vi "RunTest2.vi"(8 "error in (no error)":errorcluster, 11 "AjustesPrevios in":refnum<class "AjustesPrevios.lvclass">) -> (0 "error out":errorcluster, 2 "resultado":string, 3 "AjustesPrevios out":refnum<class "AjustesPrevios.lvclass">)   [LabVIEW 2019]
uses:
  AjustesPrevios.lvclass
  <vilib>/Utility/miscctls.llb/LVRowAndColumnTypeDef.ctl
  Controles/MessageAjustesPrev.ctl
  Prueba/Prueba.lvclass
  Controles/EstadosAjsutesPrev.ctl
  Globals/globales.vi
  Instrumento/Pistofono/Pistofono.lvclass
  QMH/User Event - Stop/User Event - Stop.lvlib
  QMH/Message Queue/Message Queue.lvlib
  QMH/Message Queue/Enqueue Message (Single).vi
  Controles/ClusterLecturaPistofono.ctl
  Controles/ClusterLecturaKeithley.ctl
  RerenceAllControlsToolkit/_get control reference by name.vi
  RerenceAllControlsToolkit/_get mutiple control reference by name.vi
  D:/REPO/GitHub/procal/Pruebas/Prueba/Prueba.lvclass
  Prueba04/Control/Slide.ctl
  Prueba04/Prueba04.lvclass
panel:
  in  "generar_CAM 2":bool
  out "Sim":bool
  out "Vguardado":dbl
  out "size_frec":i32
  in  "Tabs":enum32{"Ajustes 1", "Ajustes 2", "Ajustes 3"}(tab)
  out "factor_correccion_enviado":dbl format="%#.5g"
  in  "aplicar FC":bool
  out "Voltaje mV":dbl format="%#.3g"
  out "Nivel Medido":dbl format="%#.2g"
  out "temperatura":dbl
  out "presion":dbl
  in  "humedad":dbl
  out "nivel_emitido":dbl
  out "factor_correccion":dbl format="%#.5g"
  in  "siguiente1":bool
  in  "Sensibilidad":dbl(knob)=0.1 scale=0.01..1.0 scale format="%#_6p"
  out "voltaje a CAM":dbl format="%#_5g"
  out "frecuencia":dbl
  in  "guardar":bool
  in  "generar":bool
  in  "anterior2":bool
  in  "ajusteAmp(mV)":T1=1.0 caption="Ajuste de amplitud [V]" scale=0.1..1.5
  in  "siguiente2":bool
  in  "generar_CAM":bool
  out "voltaje":dbl format="%_3g"
  out "frecuencia":dbl
  out "NPS":dbl format="%#_4g"
  in  "anterior3":bool
  in  "terminar":bool
  out "Tabla":string[][](table)
  # "Información Pistófono"
  # "Nivel Medido [dB]"
  # "Factor de Corrección Calculado"
  # "Factor de Corrección Enviado"
  # "Voltaje [V]"
  # "Temperatura [°C]"
  # "Presión [hPa]"
  # "Humedad [%]"
  # "Nivel Emitido [dB]"
  # "Ajuste Previo 1 : Igualación de Patrones"
  # "Monitoreo"
  # "Voltaje a CAM"
  # "V"
  # "Frecuencia"
  # "Hz"
  # "Ajuste Previo 2 : Ajuste Acústico Emisor Multitono"
  # "Monitoreo"
  # "NPS"
  # "dB"
  # "Voltaje a CAM"
  # "V"
  # "Frecuencia"
  # "Hz"
  # "Ajuste Previo 3 : Niveles de Presión Sonora de Referencia"
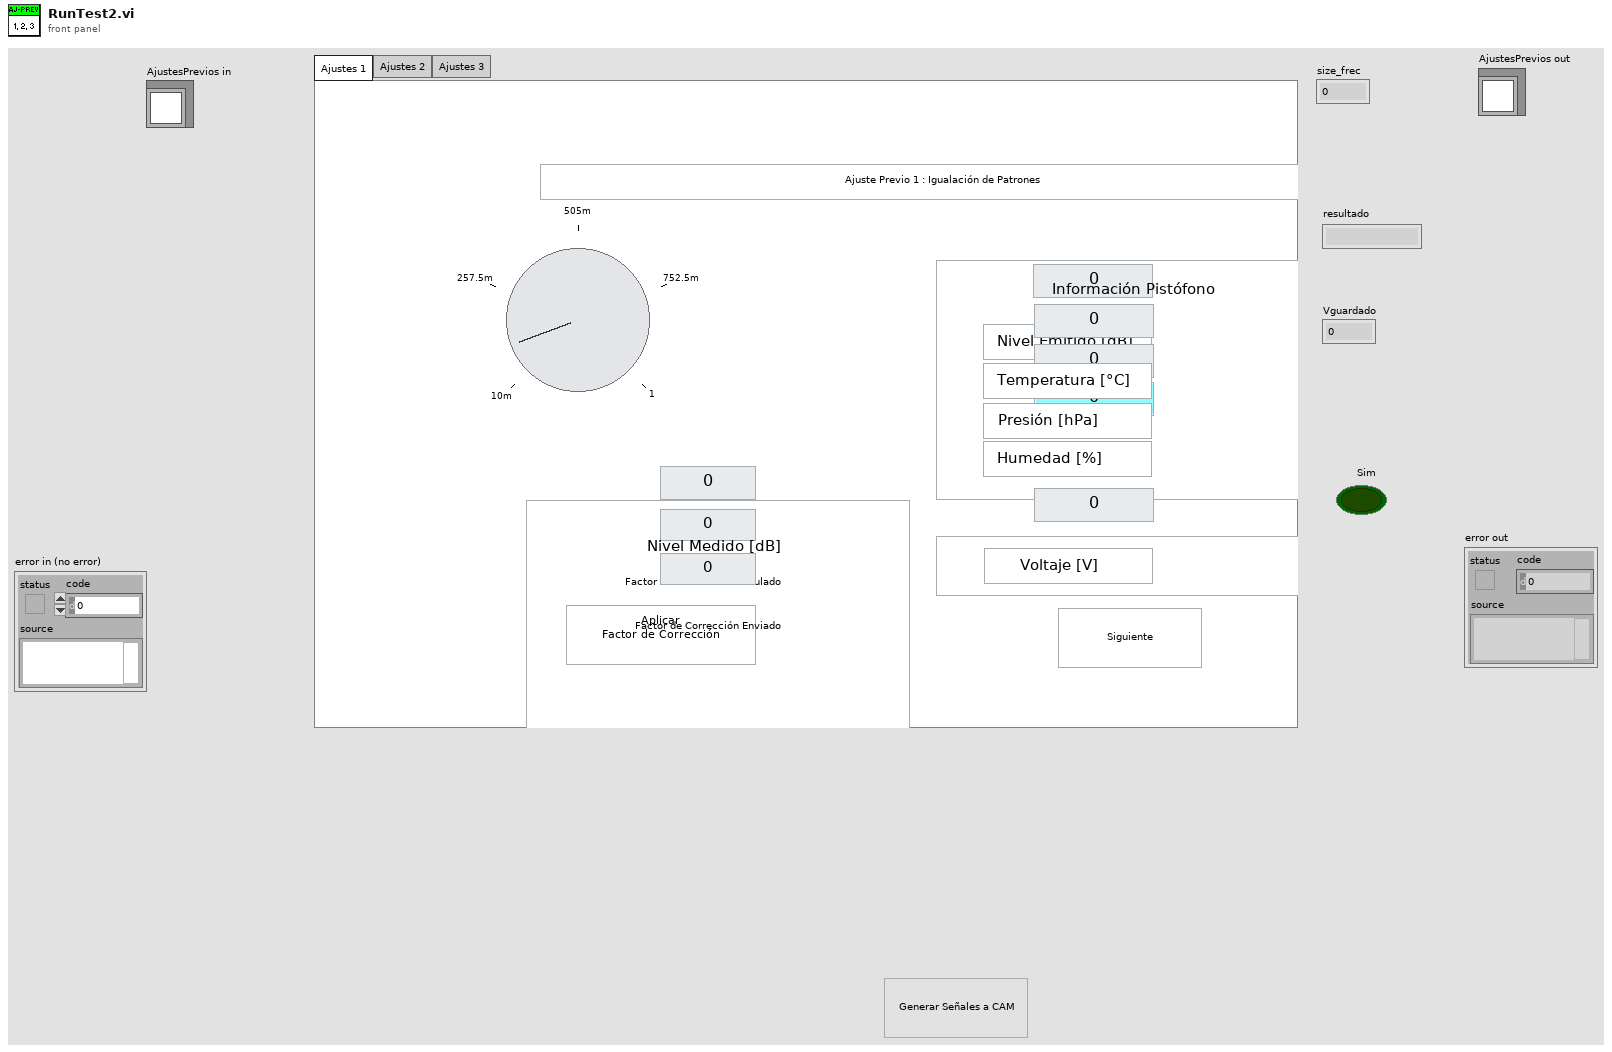
[diagram p1: front panel]
types:
  T1 = typedef "Prueba04.lvclass/Slide.ctl" = dbl
  T2 = typedef "Prueba.lvclass/MessageAjustesPrev.ctl" = cluster{"Estados":T3, "Data":variant}
  T3 = typedef "Prueba.lvclass/EstadosAjsutesPrev.ctl" = enum16{"inicio", "iniciaInstrumentos", "configurarTabla", "Ajustes1", "escribeSensib", "aplicarFC", "escribir_datos_igual_patrones", "preguntar_gen", "Ajustes2", "generar", "detenerGEN", "monitorear", "guardar", "Ajustes3", "generarCAM_94", "avisoParaCAM114", "generarCAM_114", "salir", "error", "reconec_pistofono"}
  T4 = typedef "LVRowAndColumnTypeDef.ctl" = cluster{"Row":i32, "Column":i32}
  T5 = typedef "Message Queue.lvlib/All Message Queues.ctl" = cluster{"MHL":refnum<queue>, "Inst_CNT90":refnum<queue>, "Inst_DS360":refnum<queue>, "Inst_Keithley2002":refnum<queue>, "Inst_DAQ":refnum<queue>, "BD":refnum<queue>, "Pistofono":refnum<queue>, "Nexus":refnum<queue>}
  T6 = typedef "AjustesPrevios.lvclass/ClusterLecturaPistofono.ctl" = cluster{"temperatura":dbl, "presion":dbl, "nivel_emitido":dbl}
  T7 = typedef "AjustesPrevios.lvclass/ClusterLecturaKeithley.ctl" = cluster{"Nivel_Medido_dB":dbl, "voltaje_mV":dbl}
  T8 = enum8{"Enabled", "Disabled", "Disabled and Grayed Out"}
  T9 = cluster{"ControlName":string, "ControlReference":refnum<vi>}[]
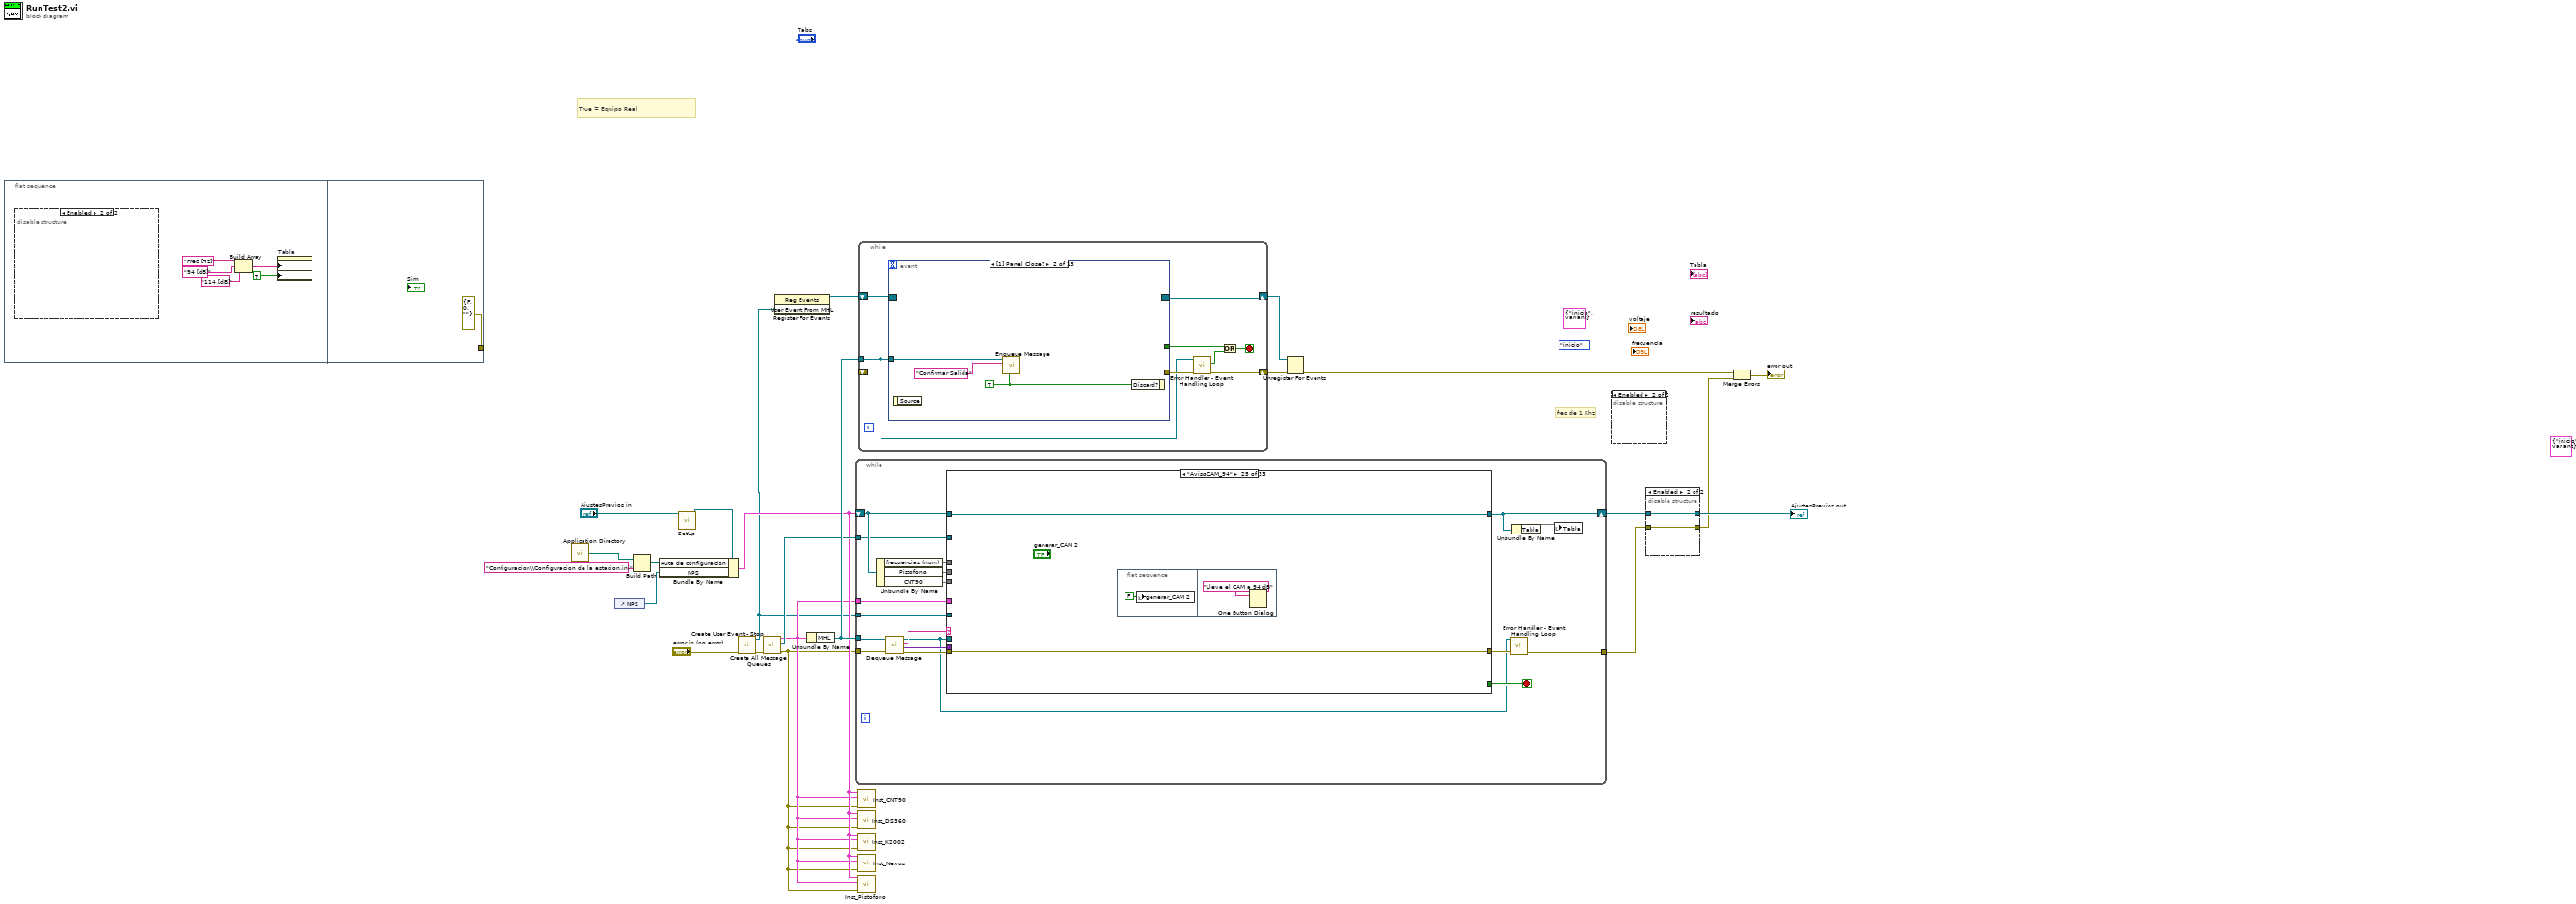
[diagram p0: block diagram]
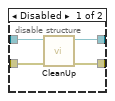
[diagram p2: hidden frame]
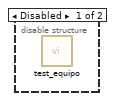
[diagram p3: hidden frame]
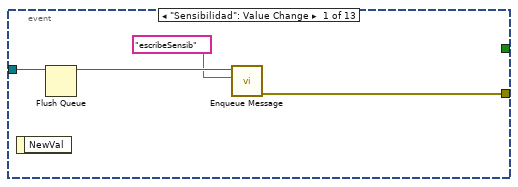
[diagram p4: hidden frame]
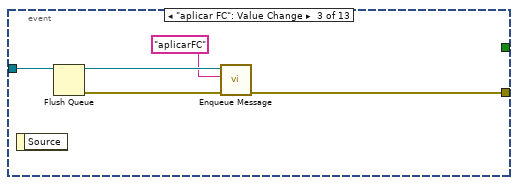
[diagram p5: hidden frame]
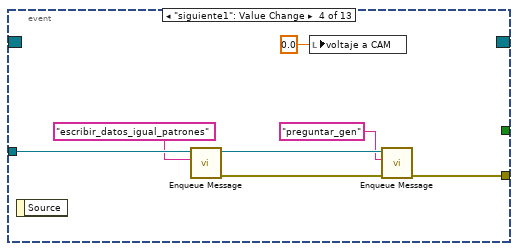
[diagram p6: hidden frame]
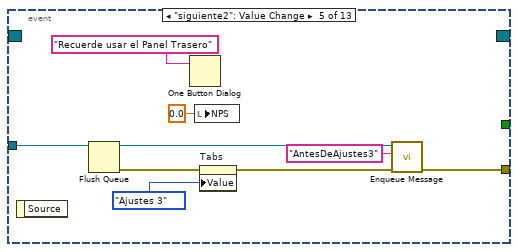
[diagram p7: hidden frame]
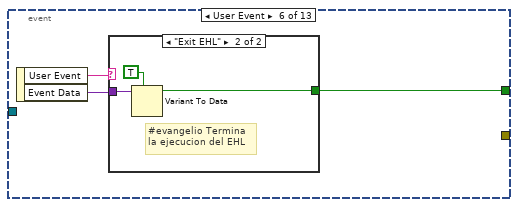
[diagram p8: hidden frame]
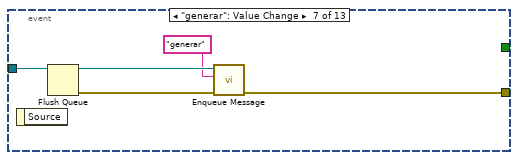
[diagram p10: hidden frame]
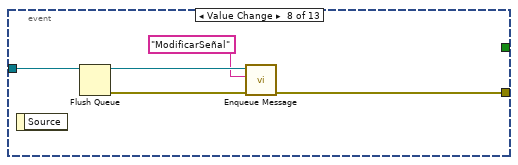
[diagram p11: hidden frame]
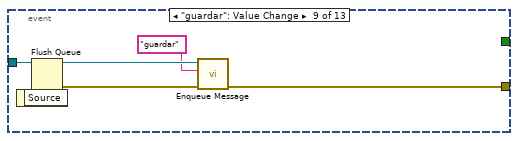
[diagram p12: hidden frame]
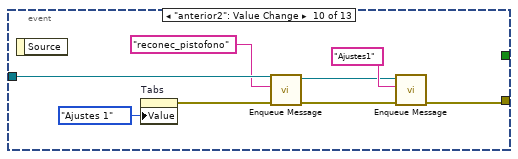
[diagram p13: hidden frame]
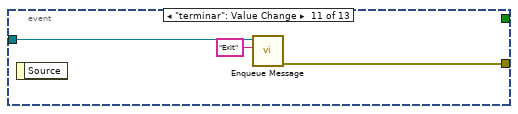
[diagram p14: hidden frame]
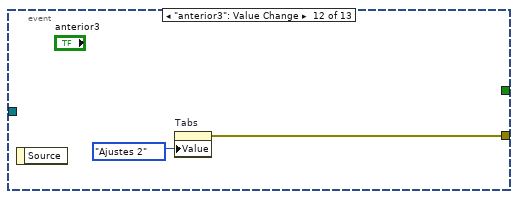
[diagram p15: hidden frame]
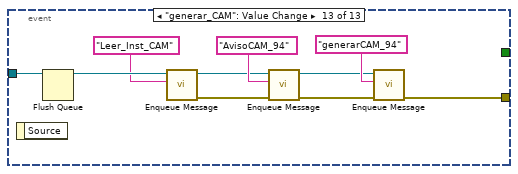
[diagram p16: hidden frame]
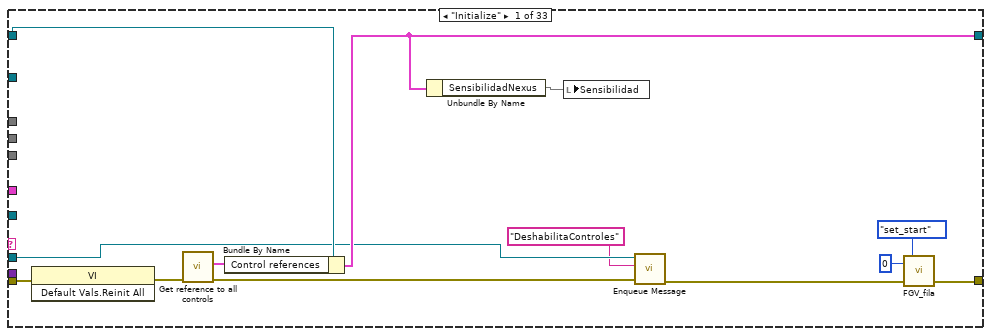
[diagram p17: hidden frame]
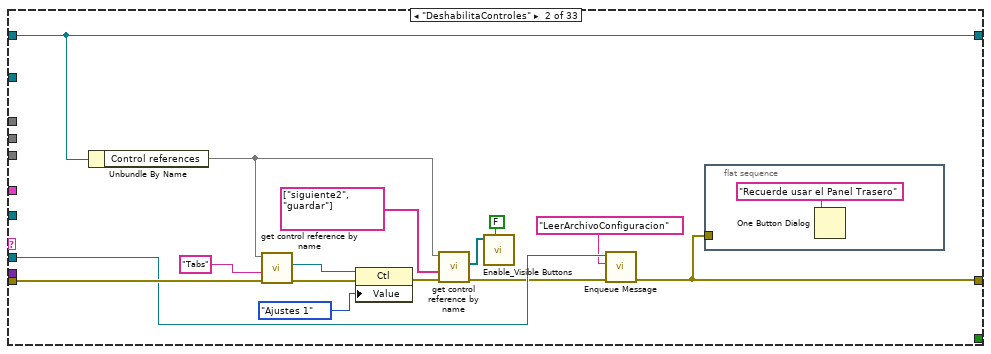
[diagram p18: hidden frame]
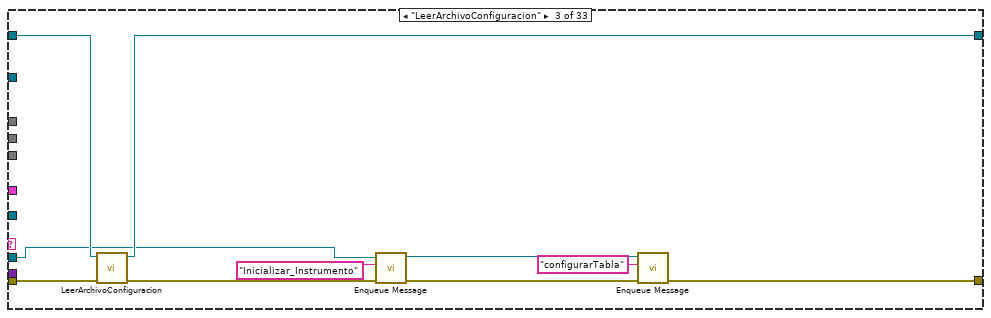
[diagram p19: hidden frame]
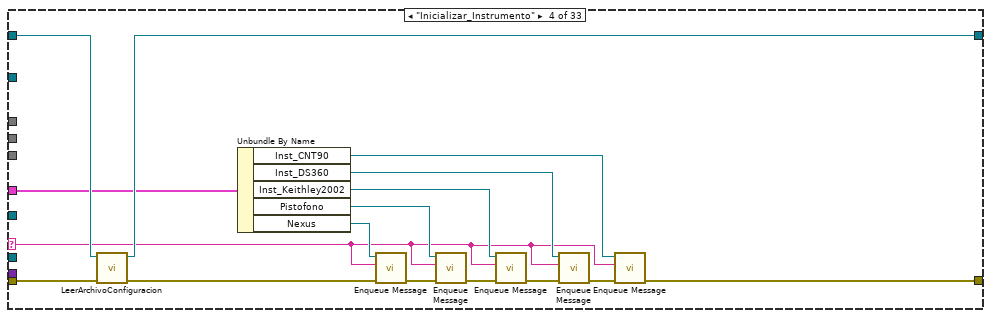
[diagram p20: hidden frame]
diagram:
  (unwired) T2 {"Estados"=enum."inicio", "Data"=variant}
  (unwired) EstadosAjsutesPrev."inicio" ("Estados")
  (unwired) T2 {"Estados"=enum."inicio", "Data"=variant}
  # "frec de 1 Khz"
  # "True = Equipo Real"
  n1 = flat-sequence {
    tunnel: [errorcluster {"status"=FALSE, "code"=0, "source"=""} ("error in (no error)")] -> _
    frame #0 {
      n2 = disable-structure shown="Enabled" {
        frame Disabled {
          n3 = Bundle By Name(cluster=T4 {"Row"=0, "Column"=0} ("Active Cell:Active Cell"), "Row"=-2, "Column"=-2) -> (w29:T4)
          n4 = property on="Tabla" class="Tbl (strict)"("Active Cell"=w29, "CellFontSize"=u32 20 ("Active Cell:Cell Font:Size"), "Justify"=enum16{"Left", "Center", "Right"}."Center" ("Active Cell:Cell Justification")) -> ()  [unwired: 2 in, 2 out]
        }
        frame Enabled {
        }
      }
    }
    frame #1 {
      n5 = Build Array("Frec [Hz]", "94 [dB]", "114 [dB]" ("element")) -> (w31:string[])
      n6 = property on="Tabla" class="Tbl (strict)"("Column Headers[]"=w31, "Col Headers Vis"=TRUE ("Visible Items:Column Headers Visible")) -> ()  [unwired: 2 in, 2 out]
    }
    frame #2 {
    }
  }
  n7 = call <vilib>:"Application Directory.vi"() -> ("Application Directory"=w13:path)
  n8 = control-ref of="NPS"() -> (w1:refnum<vi>)
  n9 = Build Path(base path=w13, name or relative path="Configuracion\\Configuracion de la estacion.ini") -> (appended path=w12:path)
  n10 = call-dynamic "SetUp.vi"("AjustesPrevios in"="AjustesPrevios in") -> ("AjustesPrevios out"=w11:refnum<class "AjustesPrevios.lvclass">)  [unwired: 9 in, 1 out]
  n11 = Bundle By Name(cluster=w11, "Ruta de configuracion"=w12, "NPS"=w1) -> (w7:cluster{})
  n12 = call "Create User Event - Stop.vi"("error in (no error)"="error in (no error)") -> ("error out"=w15:errorcluster, "User Event From MHL"=w5:refnum<user-event>)  [unwired: 9 in]
  n13 = call "Create All Message Queues.vi"("error in (no error)"=w15) -> ("error out"=w2:errorcluster, "PL Queues Array"=w8:refnum<queue>[], "All Message Queues out"=w6:T5)  [unwired: 8 in]
  n14 = register-events(w5) -> (reference out=w19:refnum<event-registration>)  [unwired: 2 in, 1 out]
  n15 = Unbundle By Name(w6) -> ("MHL"=w9:refnum<queue>)
  n16 = while {
    tunnel: w9 -> [w46]
    tunnel: w2 -> [w45]
    shift-right: [w51] -> w20
    shift-left: w7 -> [w52]
    tunnel: w6 -> [w41]
    tunnel: w8 -> [w40]
    tunnel: w5 -> [w39]
    tunnel: [w36] -> w4
    stop <- w53 stop-if-true
    n17 = Unbundle By Name(w52) -> ("frecuencias (num)"=w48, "Pistofono"=w49, "CNT90"=w47)
    n18 = call "Dequeue Message.vi"("error in (no error)"=w45, "Message Queue"=w46) -> ("error out"=w44:errorcluster, "Message Data"=w42:variant, "Message"=w43:string, "dup Message Queue"=w37:refnum<queue>)  [unwired: 6 in]
    n19 = case shown="\"AvisoCAM_94\"" w43 {
      selector: w43 -> [_ _ _ w93 w109 _ _ _ _ _ _ _ _ _ _ _ _ _ _ _ _ _ _ _ _ _ _ _ w425 _ _ _ _]
      tunnel: w44 -> [w61 w80 w91 w107 w121 w133 w136 w161 w163 w170 w179 w185 w196 w208 w212 w230 w247 w268 w270 w286 w293 w303 w305 w311 w313 w325 w370 w394 w428 w445 w454 w456 w458]
      tunnel: [w66 w67 w87 w92 w108 w123 w135 w155 w163 w167 w175 w183 w191 w205 w211 w219 w248 w264 w270 w275 w288 w299 w305 w309 w313 w337 w366 w390 w421 w439 w452 w456 w458] -> w38
      tunnel: [_ _ _ _ _ _ _ _ _ _ _ _ _ _ _ _ _ _ _ _ _ _ _ _ _ _ _ _ w423 _ _ _ _] -> w53
      tunnel: w52 -> [w59 w81 w89 w105 w120 w132 w142 w158 w162 w171 w180 w186 w194 w209 w216 w229 w239 w267 w269 w281 w289 w302 w304 w310 w312 w331 w369 w386 w424 w448 w453 w455 w457]
      tunnel: [w58 w81 w88 w104 w120 w132 w142 w156 w162 w171 w180 w186 w195 w200 w217 w237 w238 w267 w269 w281 w289 w298 w304 w310 w312 w328 w369 w383 w424 w448 w453 w455 w457] -> w51
      tunnel: w49 -> [_ _ _ _ _ _ _ _ _ _ _ _ _ _ _ _ _ _ _ _ _ _ _ _ _ _ _ _ _ _ _ _ _]
      tunnel: w48 -> [_ _ _ _ _ _ _ _ _ _ _ _ _ _ _ _ _ _ _ _ _ _ _ _ _ w334 _ w387 _ _ _ _ _]
      tunnel: w47 -> [_ _ _ _ _ _ _ _ _ _ _ _ _ _ _ _ _ _ _ _ _ _ _ _ _ _ _ _ _ _ _ _ _]
      tunnel: w37 -> [w57 w70 w86 _ _ _ w137 w153 _ _ _ _ _ _ _ _ w243 _ _ _ _ _ _ _ _ w323 w368 w373 w427 w441 _ _ _]
      tunnel: w42 -> [_ _ _ _ _ _ _ _ _ _ w178 w184 _ w207 _ _ _ _ _ _ _ _ _ _ _ _ _ _ _ w444 _ _ _]
      tunnel: w41 -> [_ _ _ w103 w119 w131 _ _ _ w169 _ _ w190 _ w215 w228 _ w266 _ w285 w292 w296 _ w308 _ w321 _ w377 _ _ w451 _ _]
      tunnel: w40 -> [_ _ _ _ _ _ _ _ _ _ _ _ _ _ _ _ _ _ _ _ _ _ _ _ _ _ _ _ w422 _ _ _ _]
      tunnel: w39 -> [_ _ _ _ _ _ _ _ _ _ _ _ _ _ _ _ _ _ _ _ _ _ _ _ _ _ _ _ w426 _ _ _ _]
      frame "Initialize" {
        n20 = invoke class="VI" method="Default Vals.Reinit All"(error in=w61) -> (error out=w62:errorcluster)  [unwired: 2 in, 2 out]
        n21 = call "Get reference to all controls.vi"("error in (no error)"=w62) -> ("error out"=w55:errorcluster, "Control references"=w60:T9)  [unwired: 5 in]
        n22 = Bundle By Name(cluster=w59, "Control references"=w60) -> (w58:cluster{})
        n23 = Unbundle By Name(w58) -> ("SensibilidadNexus"=w63)
        n24 = local write "Sensibilidad"(w63) -> ()
        n25 = call-poly "Enqueue Message.vi"("error in (no error)"=w55, "Message"="DeshabilitaControles", "Message Queue"=w57) -> ("error out"=w54:errorcluster)  [unwired: 7 in, 1 out]
        n26 = call "FGV_fila.vi"("error in (no error)"=w54, "fila_inicial"=0, "action"=enum16{"increment", "set_start", "get"}."set_start") -> ("error out"=w66:errorcluster)  [unwired: 1 in, 1 out]
      }
      frame "DeshabilitaControles" {
        n27 = Unbundle By Name(w81) -> ("Control references"=w71)
        n28 = call-poly "get control reference by name.vi"("error in (no error)"=w80, "Control name"="Tabs", "Control references"=w71) -> ("error out"=w78:errorcluster, "Ctl Refnum"=w75:refnum<vi>)  [unwired: 3 in]
        n29 = property on="Property Node" class="Ctl"(reference=w75, error in=w78, "Value"=enum32{"Ajustes 1", "Ajustes 2", "Ajustes 3"}."Ajustes 1" ("Tabs")) -> (error out=w77:errorcluster)  [unwired: 1 out]
        n30 = call-poly "get control reference by name.vi"("error in (no error)"=w77, "Control names"=string[] ["siguiente2", "guardar"] ("Control name"), "Control references"=w71) -> ("error out"=w69:errorcluster, "References"=w72:refnum<vi>[])  [unwired: 3 in]
        n31 = call "Enable_Visible Buttons.vi"("Enable? (T)"=FALSE, "Controls Ref Array"=w72) -> ()  [unwired: 10 in]
        n32 = call-poly "Enqueue Message.vi"("error in (no error)"=w69, "Message"="LeerArchivoConfiguracion", "Message Queue"=w70) -> ("error out"=w67:errorcluster)  [unwired: 7 in, 1 out]
        n33 = flat-sequence {
          tunnel: w67 -> [_]
          frame #0 {
            n34 = One Button Dialog(message="Recuerde usar el Panel Trasero") -> ()  [unwired: 1 in, 1 out]
          }
        }
      }
      frame "LeerArchivoConfiguracion" {
        n35 = call "LeerArchivoConfiguracion.vi"("error in"=w91, "AjustesPrevios in"=w89) -> ("error out"=w90:errorcluster, "AjustesPrevios out"=w88:refnum<class "AjustesPrevios.lvclass">)  [unwired: 8 in]
        n36 = call-poly "Enqueue Message.vi"("error in (no error)"=w90, "Message"="Inicializar_Instrumento", "Message Queue"=w86) -> ("error out"=w87:errorcluster, "dup Message Queue"=w84:refnum<queue>)  [unwired: 7 in]
        n37 = call-poly "Enqueue Message.vi"("Message"="configurarTabla", "Message Queue"=w84) -> ()  [unwired: 8 in, 2 out]
      }
      frame "Inicializar_Instrumento" {
        n38 = call "LeerArchivoConfiguracion.vi"("error in"=w107, "AjustesPrevios in"=w105) -> ("error out"=w106:errorcluster, "AjustesPrevios out"=w104:refnum<class "AjustesPrevios.lvclass">)  [unwired: 8 in]
        n39 = Unbundle By Name(w103) -> ("Inst_CNT90"=w98:refnum<queue>, "Inst_DS360"=w97:refnum<queue>, "Inst_Keithley2002"=w96:refnum<queue>, "Pistofono"=w95:refnum<queue>, "Nexus"=w94:refnum<queue>)
        n40 = call-poly "Enqueue Message.vi"("error in (no error)"=w106, "Message"=w93, "Message Queue"=w94) -> ("error out"=w102:errorcluster)  [unwired: 7 in, 1 out]
        n41 = call-poly "Enqueue Message.vi"("error in (no error)"=w102, "Message"=w93, "Message Queue"=w95) -> ("error out"=w101:errorcluster)  [unwired: 7 in, 1 out]
        n42 = call-poly "Enqueue Message.vi"("error in (no error)"=w101, "Message"=w93, "Message Queue"=w96) -> ("error out"=w100:errorcluster)  [unwired: 7 in, 1 out]
        n43 = call-poly "Enqueue Message.vi"("error in (no error)"=w100, "Message"=w93, "Message Queue"=w97) -> ("error out"=w99:errorcluster)  [unwired: 7 in, 1 out]
        n44 = call-poly "Enqueue Message.vi"("error in (no error)"=w99, "Message"=w93, "Message Queue"=w98) -> ("error out"=w92:errorcluster)  [unwired: 7 in, 1 out]
      }
      frame "Detener_Instrumento" {
        n45 = Unbundle By Name(w119) -> ("Inst_CNT90"=w114:refnum<queue>, "Inst_DS360"=w113:refnum<queue>, "Inst_Keithley2002"=w112:refnum<queue>, "Pistofono"=w111:refnum<queue>, "Nexus"=w110:refnum<queue>)
        n46 = call-poly "Enqueue Message.vi"("error in (no error)"=w121, "Message"=w109, "Message Queue"=w110) -> ("error out"=w118:errorcluster)  [unwired: 7 in, 1 out]
        n47 = call-poly "Enqueue Message.vi"("error in (no error)"=w118, "Message"=w109, "Message Queue"=w111) -> ("error out"=w117:errorcluster)  [unwired: 7 in, 1 out]
        n48 = call-poly "Enqueue Message.vi"("error in (no error)"=w117, "Message"=w109, "Message Queue"=w112) -> ("error out"=w116:errorcluster)  [unwired: 7 in, 1 out]
        n49 = call-poly "Enqueue Message.vi"("error in (no error)"=w116, "Message"=w109, "Message Queue"=w113) -> ("error out"=w115:errorcluster)  [unwired: 7 in, 1 out]
        n50 = call-poly "Enqueue Message.vi"("error in (no error)"=w115, "Message"=w109, "Message Queue"=w114) -> ("error out"=w108:errorcluster)  [unwired: 7 in, 1 out]
      }
      frame "Detener_Instrumento_Final" {
        w122 = "Detener_Instrumento"
        # "No consideramos el pistofono\nporque ya fue desconectado"
        n51 = Unbundle By Name(w131) -> ("Inst_CNT90"=w127:refnum<queue>, "Inst_DS360"=w126:refnum<queue>, "Inst_Keithley2002"=w125:refnum<queue>, "Nexus"=w124:refnum<queue>)  [unwired: 1 out]
        n52 = call-poly "Enqueue Message.vi"("error in (no error)"=w133, "Message"=w122, "Message Queue"=w124) -> ("error out"=w130:errorcluster)  [unwired: 7 in, 1 out]
        n53 = call-poly "Enqueue Message.vi"("error in (no error)"=w130, "Message"=w122, "Message Queue"=w125) -> ("error out"=w129:errorcluster)  [unwired: 7 in, 1 out]
        n54 = call-poly "Enqueue Message.vi"("error in (no error)"=w129, "Message"=w122, "Message Queue"=w126) -> ("error out"=w128:errorcluster)  [unwired: 7 in, 1 out]
        n55 = call-poly "Enqueue Message.vi"("error in (no error)"=w128, "Message"=w122, "Message Queue"=w127) -> ("error out"=w123:errorcluster)  [unwired: 7 in, 1 out]
      }
      frame "Confirmar Salida" {
        n56 = Two Button Dialog(message="¿Quieres cerrar la aplicación?", 1:"No" ("T button name (\"OK\")"), 2:"Si" ("T button name (\"OK\")")) -> (T button?=w138:bool)
        n57 = case shown="True" w138 {
          tunnel: w136 -> [w143 w151]
          tunnel: [w143 w146] -> w135
          tunnel: w137 -> [_ w149]
          tunnel: "Detener_Instrumento" ("Message") -> [_ w147]
          frame False {
          }
          frame True {
            n58 = call-poly "Enqueue Message.vi"("Priority Message? (F)"=TRUE, "error in (no error)"=w151, "Message"=w147, "Message Queue"=w149) -> ("error out"=w150:errorcluster, "dup Message Queue"=w145:refnum<queue>)  [unwired: 6 in]
            n59 = call-poly "Enqueue Message.vi"("error in (no error)"=w150, "Message"="Exit", "Message Queue"=w145) -> ("error out"=w146:errorcluster)  [unwired: 7 in, 1 out]
          }
        }
      }
      frame "configurarTabla" {
        n60 = call-poly "Enqueue Message.vi"("error in (no error)"=w161, "Message"="Ajustes1", "Message Queue"=w153) -> ("error out"=w155:errorcluster)  [unwired: 7 in, 1 out]
        n61 = Unbundle By Name(w158) -> ("Tabla"=w160, "frecuencias"=w154)
        n62 = call "escribeEnTabla.vi"("parametros"=w154, "col"=0, "tabla in"=w160) -> ("tabla out"=w157:string[][])  [unwired: 8 in]
        n63 = Bundle By Name(cluster=w158, "Tabla"=w157) -> (w156:cluster{})
      }
      frame "--------------------------Ajustes 1---------------------------" {
      }
      frame "Ajustes1" {
        w164 = "Leer_Instrumento" ("Message")
        n64 = Unbundle By Name(w169) -> ("Pistofono"=w166:refnum<queue>, "Inst_Keithley2002"=w165:refnum<queue>)
        n65 = call-poly "Enqueue Message.vi"("error in (no error)"=w170, "Message"=w164, "Message Queue"=w165) -> ("error out"=w168:errorcluster)  [unwired: 7 in, 1 out]
        n66 = call-poly "Enqueue Message.vi"("error in (no error)"=w168, "Message"=w164, "Message Queue"=w166) -> ("error out"=w167:errorcluster)  [unwired: 7 in, 1 out]
      }
      frame "DatoRecibidoPistofono" {
        n67 = Variant To Data(error in=w179, type=T6 {"temperatura"=0.0, "presion"=0.0, "nivel_emitido"=0.0} ("clusterPistofono"), Variant=w178) -> (data=w176:T6, error out=w175:errorcluster)
        n68 = Unbundle By Name(w176) -> ("temperatura"=→"temperatura":dbl, "presion"=→"presion":dbl, "nivel_emitido"=→"nivel_emitido":dbl)
      }
      frame "DatoRecibidoCNT90" {
        n69 = Variant To Data(error in=w185, type=0.0, Variant=w184) -> (data=→"frecuencia":dbl, error out=w183:errorcluster)
      }
      frame "aplicarFC" {
        n70 = Unbundle By Name(w190) -> ("Nexus"=w189:refnum<queue>)
        n71 = local read "factor_correccion"() -> (w188:dbl)
        "factor_correccion_enviado" <- w188
        n72 = Unbundle By Name(w194) -> ("igualacion_de_patrones"=w193)
        n73 = Bundle By Name(cluster=w193, "FactorCorreccionSensNexus"=w188) -> (w192:cluster{})
        n74 = call-poly "Enqueue Message.vi"("error in (no error)"=w196, "Message Data"=w188, "Message"="AplicarFactorCorreccion", "Message Queue"=w189) -> ("error out"=w191:errorcluster)  [unwired: 6 in, 1 out]
        n75 = Bundle By Name(cluster=w194, "igualacion_de_patrones"=w192) -> (w195:cluster{})
      }
      frame "DatoRecibidoK2002" {
        n76 = Variant To Data(error in=w208, type=T7 {"Nivel_Medido_dB"=0.0, "voltaje_mV"=0.0} ("K2002 Data Cluster"), Variant=w207) -> (data=w202:T7, error out=w206:errorcluster)
        n77 = Unbundle By Name(w202) -> ("voltaje_mV"=w198:dbl, "Nivel_Medido_dB"=w197:dbl)
        "Voltaje mV" <- w198
        "Nivel Medido" <- w197
        "voltaje a CAM" <- w198
        "NPS" <- w197
        n78 = local read "nivel_emitido"() -> (w204:dbl)
        n79 = call "FactorCorreccion.vi"("error in (no error)"=w206, "Nivel Medido"=w197, "Nivel Emitido"=w204) -> ("error out"=w205:errorcluster, "factor_correccion"=→"factor_correccion":dbl)  [unwired: 7 in]
        n80 = Bundle By Name(cluster=w209, "Voltaje enviado a CAM"=w198, "Humedad"="humedad") -> (w200:cluster{})
      }
      frame "escribeSensib" {
        n81 = local read "Sensibilidad"() -> (w210:dbl)
        n82 = Unbundle By Name(w215) -> ("Nexus"=w214:refnum<queue>)
        n83 = call-poly "Enqueue Message.vi"("error in (no error)"=w212, "Message Data"=w210, "Message"="EscribirSensibilidad", "Message Queue"=w214) -> ("error out"=w211:errorcluster)  [unwired: 6 in, 1 out]
        n84 = Bundle By Name(cluster=w216, "SensibilidadNexus"=w210) -> (w217:cluster{})
      }
      frame "escribir_datos_igual_patrones" {
        w221 = "No_Leer_Instrumento" ("Message")
        n85 = Unbundle By Name(w228) -> ("Inst_Keithley2002"=w222:refnum<queue>, "Inst_CNT90"=w224:refnum<queue>, "Inst_DS360"=w226:refnum<queue>, "Pistofono"=w227:refnum<queue>)
        n86 = call-poly "Enqueue Message.vi"("error in (no error)"=w230, "Message"="Detener_Instrumento", "Message Queue"=w227) -> ("error out"=w225:errorcluster)  [unwired: 7 in, 1 out]
        n87 = call-poly "Enqueue Message.vi"("error in (no error)"=w225, "Message"=w221, "Message Queue"=w226) -> ("error out"=w223:errorcluster)  [unwired: 7 in, 1 out]
        n88 = call-poly "Enqueue Message.vi"("error in (no error)"=w223, "Message"=w221, "Message Queue"=w224) -> ("error out"=w220:errorcluster)  [unwired: 7 in, 1 out]
        n89 = call-poly "Enqueue Message.vi"("error in (no error)"=w220, "Message"=w221, "Message Queue"=w222) -> ("error out"=w219:errorcluster)  [unwired: 7 in, 1 out]
        n90 = Unbundle By Name(w229) -> ("igualacion_de_patrones"=w236)
        n91 = local read "nivel_emitido"() -> (w235:dbl)
        n92 = local read "temperatura"() -> (w234:dbl)
        n93 = local read "humedad"() -> (w232:dbl)
        n94 = local read "presion"() -> (w233:dbl)
        n95 = Bundle By Name(cluster=w236, "Nivel Emitido Pistófono [dB]"=w235, "Temperatura interna Pistófono[ºC]"=w234, "Presión Medida Pistófono  [hPa]"=w233, "Humedad Relativa Aire [%]"=w232) -> (w231:cluster{})
        n96 = Bundle By Name(cluster=w229, "igualacion_de_patrones"=w231) -> (w237:cluster{})
      }
      frame "preguntar_gen" {
        # "Escribe en Archivo INI"
        n97 = Flush Queue(queue=w243, error in (no error)=w247) -> (queue out=w244:refnum<queue>, error out=w245:errorcluster)  [unwired: 1 out]
        n98 = call "selccionaGenerador.vi"("error in (no error)"=w245) -> ("error out"=w246:errorcluster, "Generador"=w241:string)  [unwired: 1 in]
        n99 = call "EscribirArchivoConfiguracion.vi"("error in"=w246, "TipoGenerador"=w241, "AjustesPrevios in"=w239) -> ("error out"=w242:errorcluster, "TipoGenerador out"=w240:string, "AjustesPrevios out"=w238:refnum<class "AjustesPrevios.lvclass">)  [unwired: 6 in]
        n100 = case shown="\"Externo\", Default" w240 {
          tunnel: [w250 w256] -> w248
          tunnel: w242 -> [w254 w257]
          tunnel: w244 -> [w255 _]
          frame "Interno" {
            n101 = call-poly "Enqueue Message.vi"("error in (no error)"=w254, "Message"="Detener_Instrumento", "Message Queue"=w255) -> ("error out"=w251:errorcluster, "dup Message Queue"=w252:refnum<queue>)  [unwired: 7 in]
            n102 = call-poly "Enqueue Message.vi"("error in (no error)"=w251, "Message"="Exit", "Message Queue"=w252) -> ("error out"=w250:errorcluster)  [unwired: 7 in, 1 out]
          }
          frame "Externo", Default {
            n103 = local read "ajusteAmp(mV)"() -> (w259:T1)
            n104 = property on="Tabs" class="TabCtl (strict)"(error in=w257, "Value"=enum32{"Ajustes 1", "Ajustes 2", "Ajustes 3"}."Ajustes 2" ("Tabs")) -> (error out=w256:errorcluster)  [unwired: 1 in, 1 out]
            n105 = One Button Dialog(message="Recuerde usar el Panel Delantero") -> ()  [unwired: 1 in, 1 out]
            n106 = local write "voltaje a CAM"(w259) -> ()
          }
        }
      }
      frame "AntesDeAjustes3" {
        w261 = "No_Leer_Instrumento" ("Message")
        n107 = Unbundle By Name(w266) -> ("Inst_CNT90"=w262:refnum<queue>, "Inst_Keithley2002"=w263:refnum<queue>)
        n108 = call-poly "Enqueue Message.vi"("error in (no error)"=w268, "Message"=w261, "Message Queue"=w263) -> ("error out"=w265:errorcluster)  [unwired: 7 in, 1 out]
        n109 = call-poly "Enqueue Message.vi"("error in (no error)"=w265, "Message"=w261, "Message Queue"=w262) -> ("error out"=w264:errorcluster)  [unwired: 7 in, 1 out]
      }
      frame "--------------------------Ajustes 2---------------------------" {
      }
      frame "generar" {
        w271 = "Leer_Instrumento" ("Message")
        n110 = Unbundle By Name(w281) -> ("Control references"=w280)
        n111 = call-poly "get control reference by name.vi"("error in (no error)"=w286, "Control name"="guardar", "Control references"=w280) -> ("error out"=w282:errorcluster, "Ctl Refnum"=w277:refnum<vi>)  [unwired: 3 in]
        n112 = property class="Ctl"(reference=w277, error in=w282, "DisabledEnum"=T8."Enabled" ("Disabled")) -> (error out=w278:errorcluster)  [unwired: 1 out]
        n113 = Unbundle By Name(w285) -> ("Inst_CNT90"=w272:refnum<queue>, "Inst_Keithley2002"=w273:refnum<queue>, "Inst_DS360"=w284:refnum<queue>)
        n114 = local read "ajusteAmp(mV)"() -> (w283:T1)
        n115 = call-poly "Enqueue Message.vi"("error in (no error)"=w278, "Message Data"=w283, "Message"="GenerarSeñal", "Message Queue"=w284) -> ("error out"=w275:errorcluster)  [unwired: 6 in, 1 out]
        n116 = call-poly "Enqueue Message.vi"("Message"=w271, "Message Queue"=w273) -> ()  [unwired: 8 in, 2 out]
        n117 = call-poly "Enqueue Message.vi"("Message"=w271, "Message Queue"=w272) -> ()  [unwired: 8 in, 2 out]
      }
      frame "ModificarSeñal" {
        n118 = local read "ajusteAmp(mV)"() -> (w290:T1)
        n119 = Unbundle By Name(w292) -> ("Inst_DS360"=w291:refnum<queue>)
        n120 = call-poly "Enqueue Message.vi"("error in (no error)"=w293, "Message Data"=w290, "Message"="GenerarSeñal", "Message Queue"=w291) -> ("error out"=w288:errorcluster)  [unwired: 6 in, 1 out]
      }
      frame "guardar" {
        n121 = Unbundle By Name(w296) -> ("Inst_DS360"=w295:refnum<queue>)
        n122 = property on="siguiente2" class="Bool"("DisabledEnum"=T8."Enabled" ("Disabled")) -> ()  [unwired: 2 in, 2 out]
        n123 = One Button Dialog(message="Voltaje guardado") -> ()  [unwired: 1 in, 1 out]
        n124 = call-poly "Enqueue Message.vi"("error in (no error)"=w303, "Message"="Detener_Instrumento", "Message Queue"=w295) -> ("error out"=w299:errorcluster)  [unwired: 7 in, 1 out]
        n125 = local read "voltaje a CAM"() -> (w297:dbl)
        "Vguardado" <- w297
        n126 = Bundle By Name(cluster=w302, "Voltaje enviado a CAM"=w297) -> (w298:cluster{})
        n127 = global write "globales.vi" "Vguardado"(w297) -> ()
      }
      frame "--------------------------Ajustes 3---------------------------" {
      }
      frame "Leer_Inst_CAM" {
        n128 = Unbundle By Name(w308) -> ("Inst_Keithley2002"=w307:refnum<queue>)
        n129 = call-poly "Enqueue Message.vi"("error in (no error)"=w311, "Message"="Leer_Instrumento", "Message Queue"=w307) -> ("error out"=w309:errorcluster)  [unwired: 7 in, 1 out]
      }
      frame "AvisoCAM_94" {
        n130 = flat-sequence {
          frame #0 {
            n131 = local write "generar_CAM 2"(FALSE ("generar_CAM")) -> ()
          }
          frame #1 {
            n132 = One Button Dialog(message="Lleve el CAM a 94 dB") -> ()  [unwired: 1 in, 1 out]
          }
        }
      }
      frame "generarCAM_94" {
        # "Envía set point a generador"
        n133 = call "FGV_fila.vi"("action"=enum16{"increment", "set_start", "get"}."get") -> ("fila out"=w330:i32)  [unwired: 3 in, 1 out]
        n134 = Unbundle By Name(w321) -> ("Inst_DS360"=w320:refnum<queue>)
        n135 = Array Size(array=w334) -> (size(s)=→"size_frec":i32)
        n136 = Index Array(array=w334, index=w330) -> (element=w324)
        n137 = local read "Vguardado"() -> (w318:dbl)
        n138 = local write "frecuencia"(w324) -> ()
        n139 = call-poly "Enqueue Message.vi"("error in (no error)"=w325, "Message Data"=w318, "Message"="GenerarSeñal", "Message Queue"=w320) -> ("error out"=w322:errorcluster)  [unwired: 6 in, 1 out]
        n140 = call "Time Delay"("error in (no error)"=w322, "Delay Time (s)"=2.0) -> ("error out"=w317:errorcluster)  [unwired: 9 in]
        n141 = while {
          tunnel: w317 -> [w361]
          tunnel: [w361] -> w339
          tunnel: w331 -> [w355]
          tunnel: w330 -> [w357]
          tunnel: [w356] -> w329
          tunnel: [w355] -> w327
          i -> [w364]
          stop <- w362 stop-if-true
          # "col"
          n142 = Unbundle By Name(w355) -> ("Tabla"=w359)
          n143 = local read "NPS"() -> (w354:dbl)
          n144 = local write "generar_CAM"(TRUE ("generar_CAM")) -> ()
          n145 = Greater?(x=w364, y=2) -> (0:w362:bool)
          n146 = call "escribeEnTablaUnValor.vi"("element"=w354, "fila"=w357, "col"=1, "tabla in"=w359) -> ("tabla out"=w356:string[][])  [unwired: 7 in]
          n147 = Wait (ms)(milliseconds to wait=u32 1000) -> ()  [unwired: 1 out]
        }
        n148 = local read "size_frec"() -> (w332:i32)
        n149 = call "FGV_fila.vi"("error in (no error)"=w339, "action"=enum16{"increment", "set_start", "get"}."increment") -> ("error out"=w338:errorcluster, "fila out"=w335:i32)  [unwired: 2 in]
        n150 = Bundle By Name(cluster=w327, "Tabla"=w329) -> (w328:cluster{})
        n151 = Greater Or Equal?(x=w335, y=w332) -> (x >= y?=w336:bool)
        n152 = local read "Vguardado"() -> (w326:dbl)
        n153 = case shown="True" w336 {
          tunnel: w338 -> [w346 w353]
          tunnel: [w345 w352] -> w337
          tunnel: w323 -> [w342 w347]
          frame False {
            n154 = local write "generar_CAM"(FALSE ("generar_CAM")) -> ()
            n155 = call-poly "Enqueue Message.vi"("error in (no error)"=w346, "Message"="generarCAM_94", "Message Queue"=w342) -> ("error out"=w345:errorcluster)  [unwired: 7 in, 1 out]
          }
          frame True {
            n156 = local write "NPS"(0.0 ("NPS")) -> ()
            n157 = call "FGV_fila.vi"("fila_inicial"=0, "action"=enum16{"increment", "set_start", "get"}."set_start") -> ()  [unwired: 2 in, 2 out]
            n158 = call-poly "Enqueue Message.vi"("error in (no error)"=w353, "Message"="avisoParaCAM114", "Message Queue"=w347) -> ("error out"=w352:errorcluster)  [unwired: 7 in, 1 out]
          }
        }
        n159 = local write "voltaje"(w326) -> ()
      }
      frame "avisoParaCAM114" {
        n160 = call-poly "Enqueue Message.vi"("error in (no error)"=w370, "Message"="generarCAM_114", "Message Queue"=w368) -> ("error out"=w366:errorcluster)  [unwired: 7 in, 1 out]
        n161 = flat-sequence {
          tunnel: w366 -> [_]
          frame #0 {
            n162 = local write "generar_CAM"(FALSE ("generar_CAM")) -> ()
            n163 = One Button Dialog(message="Lleve el CAM a 114 dB") -> ()  [unwired: 1 in, 1 out]
          }
        }
      }
      frame "generarCAM_114" {
        n164 = call "FGV_fila.vi"("action"=enum16{"increment", "set_start", "get"}."get") -> ("fila out"=w385:i32)  [unwired: 3 in, 1 out]
        n165 = local read "Vguardado"() -> (w375:dbl)
        n166 = Index Array(array=w387, index=w385) -> (element=w379)
        n167 = Unbundle By Name(w377) -> ("Inst_DS360"=w374:refnum<queue>)
        n168 = local write "frecuencia"(w379) -> ()
        n169 = call-poly "Enqueue Message.vi"("error in (no error)"=w394, "Message Data"=w375, "Message"="GenerarSeñal", "Message Queue"=w374) -> ("error out"=w378:errorcluster)  [unwired: 6 in, 1 out]
        n170 = while {
          tunnel: w378 -> [w416]
          tunnel: [w416] -> w392
          tunnel: w386 -> [w410]
          tunnel: w385 -> [w412]
          tunnel: [w411] -> w384
          tunnel: [w410] -> w382
          i -> [w419]
          stop <- w417 stop-if-true
          # "col"
          n171 = Unbundle By Name(w410) -> ("Tabla"=w414)
          n172 = local write "generar_CAM"(TRUE ("generar_CAM")) -> ()
          n173 = local read "NPS"() -> (w409:dbl)
          n174 = Greater?(x=w419, y=2) -> (0:w417:bool)
          n175 = call "escribeEnTablaUnValor.vi"("element"=w409, "fila"=w412, "col"=2, "tabla in"=w414) -> ("tabla out"=w411:string[][])  [unwired: 7 in]
          n176 = Wait (ms)(milliseconds to wait=u32 1000) -> ()  [unwired: 1 out]
        }
        n177 = local read "size_frec"() -> (w381:i32)
        n178 = call "FGV_fila.vi"("error in (no error)"=w392, "action"=enum16{"increment", "set_start", "get"}."increment") -> ("error out"=w391:errorcluster, "fila out"=w388:i32)  [unwired: 2 in]
        n179 = Bundle By Name(cluster=w382, "Tabla"=w384) -> (w383:cluster{})
        n180 = Greater Or Equal?(x=w388, y=w381) -> (x >= y?=w389:bool)
        n181 = case shown="True" w389 {
          tunnel: w391 -> [w400 w408]
          tunnel: [w399 w403] -> w390
          tunnel: w373 -> [w396 w402]
          frame False {
            n182 = local write "generar_CAM"(FALSE ("generar_CAM")) -> ()
            n183 = call-poly "Enqueue Message.vi"("error in (no error)"=w400, "Message"="generarCAM_114", "Message Queue"=w396) -> ("error out"=w399:errorcluster)  [unwired: 7 in, 1 out]
          }
          frame True {
            n184 = call "FGV_fila.vi"("fila_inicial"=0, "action"=enum16{"increment", "set_start", "get"}."set_start") -> ()  [unwired: 2 in, 2 out]
            n185 = One Button Dialog(message="Generación de frecuencias OK") -> ()  [unwired: 1 in, 1 out]
            n186 = local write "generar_CAM"(FALSE) -> ()
            n187 = call-poly "Enqueue Message.vi"("error in (no error)"=w408, "Message"="Detener_Instrumento_Final", "Message Queue"=w402) -> ("error out"=w403:errorcluster)  [unwired: 7 in, 1 out]
          }
        }
        n188 = local read "Vguardado"() -> (w380:dbl)
        n189 = local write "voltaje"(w380) -> ()
      }
      frame "Exit" {
        w423 = TRUE
        # "#evangelio Manda a cerrar el EHL"
        # "#evangelio Manda a cerrar todos los Loops"
        n190 = Release Queue(queue=w427, error in (no error)=w428) -> (error out=w432:errorcluster)  [unwired: 1 in, 2 out]
        n191 = Unbundle By Name(w424) -> ("Control references"=w433)
        n192 = for {
          tunnel: w422 -> [w436] mode=indexing
          tunnel: w425 -> [w435]
          tunnel: TRUE -> [w434]
          n193 = call-poly "Enqueue Message.vi"("Priority Message? (F)"=w434, "Message"=w435, "Message Queue"=w436) -> ()  [unwired: 7 in, 2 out]
        }
        n194 = call "Close All Ref.vi"("error in (no error)"=w432, "Control references"=w433) -> ("error out"=w430:errorcluster)  [unwired: 9 in]
        n195 = call "Fire User Event - Stop.vi"("error in (no error)"=w430, "Event Data"=w423, "User Event"="Exit EHL", "User Event in"=w426) -> ("error out"=w421:errorcluster)  [unwired: 7 in]
      }
      frame "Error" {
        n196 = Variant To Data(error in=w445, type=errorcluster {"status"=FALSE, "code"=0, "source"=""} ("error constant"), Variant=w444) -> (data=w446:errorcluster, error out=w443:errorcluster)
        n197 = call <vilib>:"Simple Error Handler.vi"("error in (no error)"=w446) -> ()  [unwired: 4 in, 5 out]
        n198 = call-poly "Enqueue Message.vi"("error in (no error)"=w443, "Message"="Detener_Instrumento", "Message Queue"=w441) -> ("error out"=w442:errorcluster, "dup Message Queue"=w438:refnum<queue>)  [unwired: 7 in]
        n199 = call-poly "Enqueue Message.vi"("error in (no error)"=w442, "Message"="Exit", "Message Queue"=w438) -> ("error out"=w439:errorcluster)  [unwired: 7 in, 1 out]
      }
      frame "reconec_pistofono" {
        n200 = Unbundle By Name(w451) -> ("Pistofono"=w450:refnum<queue>)
        n201 = call-poly "Enqueue Message.vi"("error in (no error)"=w454, "Message"="Inicializar_Instrumento", "Message Queue"=w450) -> ("error out"=w452:errorcluster)  [unwired: 7 in, 1 out]
      }
      frame Default {
      }
      frame "--------------------------Controles---------------------------" {
      }
    }
    n202 = call "Error Handler - Event Handling Loop.vi"("error in (no error)"=w38, "Message Queue"=w37) -> ("dup error in"=w36:errorcluster)  [unwired: 7 in, 2 out]
    n203 = Unbundle By Name(w51) -> ("Tabla"=w50)
    n204 = local write "Tabla"(w50) -> ()
  }
  n205 = call "Inst_CNT90.vi"("error in"=w2, "All Message Queues in"=w6, "AjustesPrevios in"=w7) -> ()  [unwired: 8 in, 1 out]
  n206 = call "Inst_DS360.vi"("error in"=w2, "All Message Queues in"=w6, "AjustesPrevios in"=w7) -> ()  [unwired: 8 in, 1 out]
  n207 = call "Inst_K2002.vi"("error in"=w2, "All Message Queues in"=w6, "AjustesPrevios in"=w7) -> ()  [unwired: 8 in, 1 out]
  n208 = call "Inst_Nexus.vi"("error in"=w2, "All Message Queues in"=w6, "AjustesPrevios in"=w7) -> ()  [unwired: 8 in, 1 out]
  n209 = call "Inst_Pistofono.vi"("error in"=w2, "All Message Queues in"=w6, "AjustesPrevios in"=w7) -> ()  [unwired: 8 in, 1 out]
  n210 = while {
    tunnel: w9 -> [w461]
    shift-right: [w465] -> w17
    shift-left: w19 -> [w466]
    shift-right: [w462] -> w22
    shift-left: _ -> [_]
    stop <- w463 stop-if-true
    n211 = event shown="[1] Panel Close?" {
      selector: w466 -> [_ _ _ _ _ _ _ _ _ _ _ _ _]
      dyn-events: [_ _ _ _ _ _ _ _ _ _ _ _ _] -> w465
      timeout: _ -> [_ _ _ _ _ _ _ _ _ _ _ _ _]
      tunnel: w461 -> [w470 w472 w477 w485 w490 _ w503 w508 w513 w518 w525 _ w538]
      tunnel: [w468 _ w476 w481 w488 _ w505 w510 w515 w521 w526 w527 _] -> w464
      tunnel: [_ _ _ _ _ w495 _ _ _ _ _ _ _] -> w460
      tunnel: [_ _ _ _ _ _ _ _ _ _ _ _ w529] -> _
      event "Sensibilidad": Value Change {
        n212 = event-data() -> ()  [unwired: 1 in, 1 out]
        n213 = Flush Queue(queue=w470) -> (queue out=w469:refnum<queue>)  [unwired: 1 in, 2 out]
        n214 = call-poly "Enqueue Message.vi"("Message"="escribeSensib", "Message Queue"=w469) -> ("error out"=w468:errorcluster)  [unwired: 8 in, 1 out]
      }
      event Panel Close? {
        w471 = TRUE
        n215 = event-data() -> ()  [unwired: 1 in, 1 out]
        n216 = call-poly "Enqueue Message.vi"("Priority Message? (F)"=w471, "Message"="Confirmar Salida", "Message Queue"=w472) -> ()  [unwired: 7 in, 2 out]
        n217 = event-data("Discard?"=w471) -> ()  [unwired: 1 in, 1 out]
      }
      event "aplicar FC": Value Change {
        n218 = event-data() -> ()  [unwired: 1 in, 1 out]
        n219 = Flush Queue(queue=w477) -> (queue out=w475:refnum<queue>, error out=w478:errorcluster)  [unwired: 1 in, 1 out]
        n220 = call-poly "Enqueue Message.vi"("error in (no error)"=w478, "Message"="aplicarFC", "Message Queue"=w475) -> ("error out"=w476:errorcluster)  [unwired: 7 in, 1 out]
      }
      event "siguiente1": Value Change {
        n221 = event-data() -> ()  [unwired: 1 in, 1 out]
        n222 = call-poly "Enqueue Message.vi"("Message"="escribir_datos_igual_patrones", "Message Queue"=w485) -> ("error out"=w482:errorcluster, "dup Message Queue"=w483:refnum<queue>)  [unwired: 8 in]
        n223 = local write "voltaje a CAM"(0.0 ("NPS")) -> ()
        n224 = call-poly "Enqueue Message.vi"("error in (no error)"=w482, "Message"="preguntar_gen", "Message Queue"=w483) -> ("error out"=w481:errorcluster)  [unwired: 7 in, 1 out]
      }
      event "siguiente2": Value Change {
        n225 = event-data() -> ()  [unwired: 1 in, 1 out]
        n226 = Flush Queue(queue=w490) -> (queue out=w487:refnum<queue>, error out=w491:errorcluster)  [unwired: 1 in, 1 out]
        n227 = One Button Dialog(message="Recuerde usar el Panel Trasero") -> ()  [unwired: 1 in, 1 out]
        n228 = local write "NPS"(0.0 ("NPS")) -> ()
        n229 = property on="Tabs" class="TabCtl (strict)"(error in=w491, "Value"=enum32{"Ajustes 1", "Ajustes 2", "Ajustes 3"}."Ajustes 3" ("Tabs")) -> (error out=w493:errorcluster)  [unwired: 1 in, 1 out]
        n230 = call-poly "Enqueue Message.vi"("error in (no error)"=w493, "Message"="AntesDeAjustes3", "Message Queue"=w487) -> ("error out"=w488:errorcluster)  [unwired: 7 in, 1 out]
      }
      event User Event {
        n231 = event-data() -> ("User Event"=w497:string, "Event Data"=w496:variant)  [unwired: 1 in]
        n232 = case shown="\"Exit EHL\"" w497 {
          tunnel: w496 -> [_ w499]
          tunnel: [_ w498] -> w495
          frame Default {
          }
          frame "Exit EHL" {
            # "#evangelio Termina\nla ejecucion del EHL"
            n233 = Variant To Data(type=TRUE, Variant=w499) -> (data=w498:bool)  [unwired: 1 in, 1 out]
          }
        }
      }
      event "generar": Value Change {
        n234 = event-data() -> ()  [unwired: 1 in, 1 out]
        n235 = Flush Queue(queue=w503) -> (queue out=w502:refnum<queue>, error out=w504:errorcluster)  [unwired: 1 in, 1 out]
        n236 = call-poly "Enqueue Message.vi"("error in (no error)"=w504, "Message"="generar", "Message Queue"=w502) -> ("error out"=w505:errorcluster)  [unwired: 7 in, 1 out]
      }
      event Value Change {
        n237 = event-data() -> ()  [unwired: 1 in, 1 out]
        n238 = Flush Queue(queue=w508) -> (queue out=w507:refnum<queue>, error out=w509:errorcluster)  [unwired: 1 in, 1 out]
        n239 = call-poly "Enqueue Message.vi"("error in (no error)"=w509, "Message"="ModificarSeñal", "Message Queue"=w507) -> ("error out"=w510:errorcluster)  [unwired: 7 in, 1 out]
      }
      event "guardar": Value Change {
        n240 = event-data() -> ()  [unwired: 1 in, 1 out]
        n241 = Flush Queue(queue=w513) -> (queue out=w512:refnum<queue>, error out=w514:errorcluster)  [unwired: 1 in, 1 out]
        n242 = call-poly "Enqueue Message.vi"("error in (no error)"=w514, "Message"="guardar", "Message Queue"=w512) -> ("error out"=w515:errorcluster)  [unwired: 7 in, 1 out]
      }
      event "anterior2": Value Change {
        n243 = event-data() -> ()  [unwired: 1 in, 1 out]
        n244 = property on="Tabs" class="TabCtl (strict)"("Value"=enum32{"Ajustes 1", "Ajustes 2", "Ajustes 3"}."Ajustes 1" ("Tabs")) -> (error out=w522:errorcluster)  [unwired: 2 in, 1 out]
        n245 = call-poly "Enqueue Message.vi"("error in (no error)"=w522, "Message"="reconec_pistofono", "Message Queue"=w518) -> ("error out"=w519:errorcluster, "dup Message Queue"=w517:refnum<queue>)  [unwired: 7 in]
        n246 = call-poly "Enqueue Message.vi"("error in (no error)"=w519, "Message"="Ajustes1", "Message Queue"=w517) -> ("error out"=w521:errorcluster)  [unwired: 7 in, 1 out]
      }
      event "terminar": Value Change {
        n247 = event-data() -> ()  [unwired: 1 in, 1 out]
        n248 = call-poly "Enqueue Message.vi"("Message"="Exit", "Message Queue"=w525) -> ("error out"=w526:errorcluster)  [unwired: 8 in, 1 out]
      }
      event "anterior3": Value Change {
        n249 = event-data() -> ()  [unwired: 1 in, 1 out]
        n250 = property on="Tabs" class="TabCtl (strict)"("Value"=enum32{"Ajustes 1", "Ajustes 2", "Ajustes 3"}."Ajustes 2" ("Tabs")) -> (error out=w527:errorcluster)  [unwired: 2 in, 1 out]
      }
      event "generar_CAM": Value Change {
        n251 = event-data() -> ()  [unwired: 1 in, 1 out]
        n252 = Flush Queue(queue=w538) -> (queue out=w537:refnum<queue>)  [unwired: 1 in, 2 out]
        n253 = call-poly "Enqueue Message.vi"("Message"="Leer_Inst_CAM", "Message Queue"=w537) -> ("error out"=w532:errorcluster, "dup Message Queue"=w533:refnum<queue>)  [unwired: 8 in]
        n254 = call-poly "Enqueue Message.vi"("error in (no error)"=w532, "Message"="AvisoCAM_94", "Message Queue"=w533) -> ("error out"=w530:errorcluster, "dup Message Queue"=w531:refnum<queue>)  [unwired: 7 in]
        n255 = call-poly "Enqueue Message.vi"("error in (no error)"=w530, "Message"="generarCAM_94", "Message Queue"=w531) -> ("error out"=w529:errorcluster)  [unwired: 7 in, 1 out]
      }
    }
    n256 = call "Error Handler - Event Handling Loop.vi"("error in (no error)"=w464, "Message Queue"=w461) -> ("dup error in"=w462:errorcluster, "Error?"=w459:bool)  [unwired: 7 in, 1 out]
    n257 = Or(x=w460, y=w459) -> (x .or. y?=w463:bool)
  }
  n258 = Unregister For Events(event registration refnum=w17, error in=w22) -> (error out=w18:errorcluster)
  n259 = disable-structure shown="Enabled" {
    frame Disabled {
      n260 = call "test_equipo.vi"() -> ()  [unwired: 12 in]
    }
    frame Enabled {
    }
  }
  n261 = disable-structure shown="Enabled" {
    disable-tunnel: w20 -> [w542 w544]
    disable-tunnel: [w541 w544] -> w16
    disable-tunnel: w4 -> [w540 w543]
    disable-tunnel: [w539 w543] -> w3
    frame Disabled {
      n262 = call-dynamic "CleanUp.vi"("error in (no error)"=w540, "AjustesPrevios in"=w542) -> ("error out"=w539:errorcluster, "AjustesPrevios out"=w541:refnum<class "AjustesPrevios.lvclass">)  [unwired: 8 in]
    }
    frame Enabled {
    }
  }
  "AjustesPrevios out" <- w16
  n263 = Merge Errors(w18, w3) -> (→"error out":errorcluster)
